vi "Kinect - Control Cluster (SubVI).vi"(7 "error in":errorcluster, 8 "Calibrate Pitch":bool, 9 "Weak detect":bool, 10 "Array of Joint Positions in":dbl[][](array[numeric])=[[-0.1347254365682602, -0.08132069557905197, 1.9283822774887085], [-0.13885043561458588, -0.016961583867669106, 2.011981248855591], [-0.14481712877750397, 0.43931880593299866, 2.1406660079956055], [-0.141028493642807, 0.6465446352958679, 2.1821846961975098], [-0.30089935660362244, 0.32630765438079834, 2.0420639514923096], [-0.26517531275749207, 0.1817575842142105, 1.7472813129425049], [-0.12027974426746368, 0.18339265882968903, 1.4648816585540771], [-0.08502443134784698, 0.17742732167243958, 1.430349588394165], [-0.003267590655013919, 0.3257020115852356, 2.05509090423584], [0.025156527757644653, 0.16852739453315735, 1.7666873931884766], [-0.0971737802028656, 0.17441977560520172, 1.473292350769043], [-0.1705384999513626, 0.18324872851371765, 1.465440034866333], [-0.21323969960212708, -0.14314982295036316, 1.8959753513336182], [-0.2711157202720642, -0.4896538555622101, 1.8643081188201904], [-0.25042033195495605, -0.8901764750480652, 1.868118405342102], [-0.23817336559295654, -0.9496505260467529, 1.7813631296157837], [-0.05292607098817825, -0.14255109429359436, 1.9082472324371338], [-0.03935781121253967, -0.4929194450378418, 1.869278073310852], [-0.03272760659456253, -0.8968366384506226, 1.8476512432098389], [-0.02717301808297634, -0.9465184211730957, 1.7542997598648071]]) -> (0 "error out":errorcluster, 2 "Control Cluster out":T1={"Roll"=0.09503769, "Pitch"=0.11711881, "Vertical Speed"=0.0, "Yaw Speed"=-0.05722916} {"Yaw Speed" scale=-1.0..1.0; "Vertical Speed" scale=-1.0..1.0; "Pitch" scale=-1.0..1.0; "Roll" scale=-1.0..1.0}, 3 "Array of Joint Positions out":dbl[][](array[numeric])=[[-0.1347254365682602, -0.08132069557905197, 1.9283822774887085], [-0.13885043561458588, -0.016961583867669106, 2.011981248855591], [-0.14481712877750397, 0.43931880593299866, 2.1406660079956055], [-0.141028493642807, 0.6465446352958679, 2.1821846961975098], [-0.30089935660362244, 0.32630765438079834, 2.0420639514923096], [-0.26517531275749207, 0.1817575842142105, 1.7472813129425049], [-0.12027974426746368, 0.18339265882968903, 1.4648816585540771], [-0.08502443134784698, 0.17742732167243958, 1.430349588394165], [-0.003267590655013919, 0.3257020115852356, 2.05509090423584], [0.025156527757644653, 0.16852739453315735, 1.7666873931884766], [-0.0971737802028656, 0.17441977560520172, 1.473292350769043], [-0.1705384999513626, 0.18324872851371765, 1.465440034866333], [-0.21323969960212708, -0.14314982295036316, 1.8959753513336182], [-0.2711157202720642, -0.4896538555622101, 1.8643081188201904], [-0.25042033195495605, -0.8901764750480652, 1.868118405342102], [-0.23817336559295654, -0.9496505260467529, 1.7813631296157837], [-0.05292607098817825, -0.14255109429359436, 1.9082472324371338], [-0.03935781121253967, -0.4929194450378418, 1.869278073310852], [-0.03272760659456253, -0.8968366384506226, 1.8476512432098389], [-0.02717301808297634, -0.9465184211730957, 1.7542997598648071]])   [LabVIEW 2014]
uses:
  Resources/Others/Control cluster.ctl
panel:
  out "vertical speed":dbl(knob)=-0.14245328307151794 scale=-20.0..20.0
  in  "pitch offset":dbl=0.15 format="%#_13g"
  in  "roll adjust":dbl=1.5 format="%#_13g"
  # "Experiment-based values:"
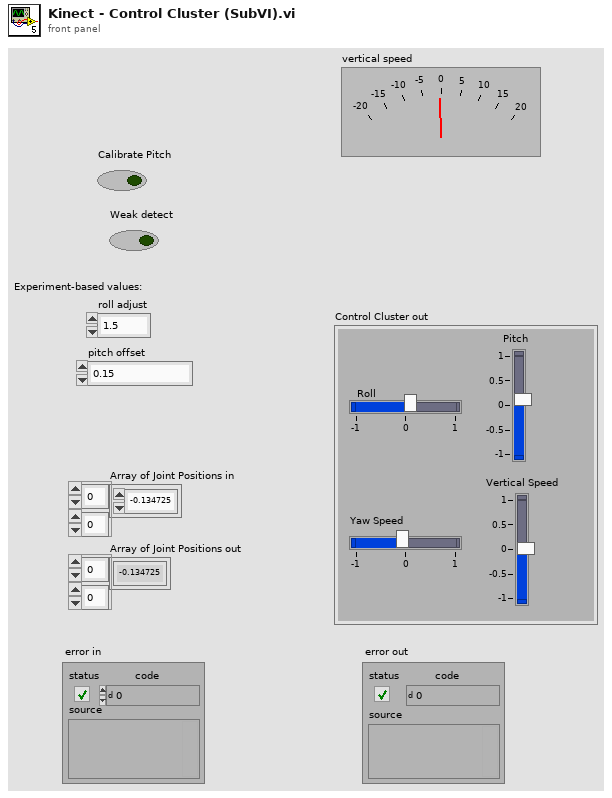
[diagram p1: front panel]
types:
  T1 = typedef "Control cluster.ctl" = cluster{"Roll":sgl, "Pitch":sgl, "Vertical Speed":sgl, "Yaw Speed":sgl}
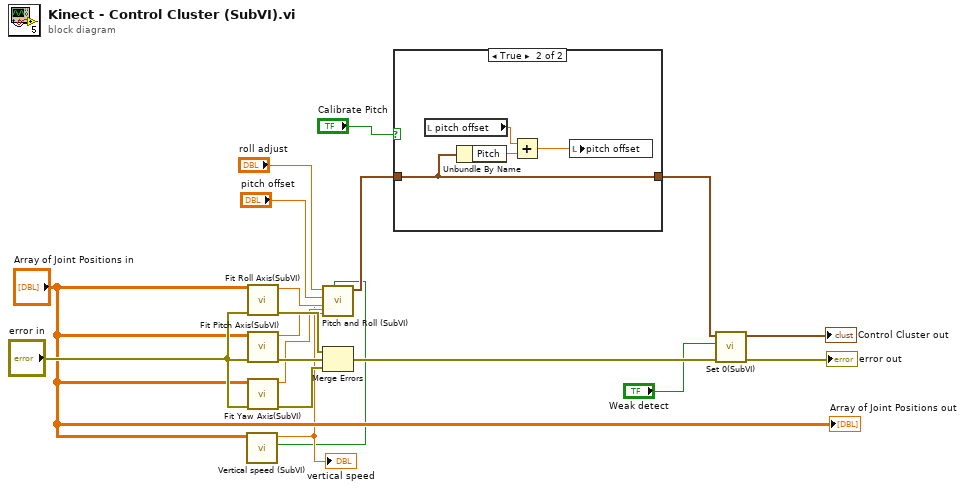
[diagram p0: block diagram]
diagram:
  n1 = call "Vertical speed (SubVI).vi"("Array of Joint Positions in"="Array of Joint Positions in") -> ("x .and. y?"=w1:bool, "Vertical Speed"=w2:dbl)  [unwired: 9 in]
  "vertical speed" <- w2
  n2 = call "Fit Roll Axis(SubVI).vi"("error in (no error)"="error in", "Array of Joint Positions in"="Array of Joint Positions in") -> ("error out"=w18:errorcluster, "slope"=w19:dbl)  [unwired: 8 in]
  n3 = call "Fit Pitch Axis(SubVI).vi"("error in (no error)"="error in", "Array of Joint Positions in"="Array of Joint Positions in") -> ("error out"=w17:errorcluster, "slope"=w16:dbl)  [unwired: 8 in]
  n4 = call "Fit Yaw Axis(SubVI).vi"("error in (no error)"="error in", "Array of Joint Positions in in"="Array of Joint Positions in") -> ("error out"=w11:errorcluster, "slope"=w12:dbl)  [unwired: 8 in]
  n5 = call "Pitch and Roll (SubVI).vi"("Vertical Speed"=w2, "yaw"=w12, "Vertical movement"=w1, "pitch"=w16, "roll"=w19, "pitch offset"="pitch offset", "roll adjust"="roll adjust") -> ("Control Cluster out"=w5:T1)  [unwired: 2 in]
  n6 = Merge Errors(w18, w17, w11) -> (w10:errorcluster)
  n7 = case shown="True" "Calibrate Pitch" {
    tunnel: w5 -> [w20 w24]
    tunnel: [w20 w24] -> w4
    frame False {
    }
    frame True {
      n8 = local read "pitch offset"() -> (w23:dbl)
      n9 = Unbundle By Name(w24) -> ("Pitch"=w22:sgl)
      n10 = Add(x=w23, y=w22) -> (x+y=w21:dbl)
      n11 = local write "pitch offset"(w21) -> ()
    }
  }
  n12 = call "Set 0(SubVI).vi"("error in (no error)"=w10, "Weak detect"="Weak detect", "Control Cluster in"=w4) -> ("error out"=→"error out":errorcluster, "Control Cluster out"=→"Control Cluster out":T1)  [unwired: 7 in]
  "Array of Joint Positions out" <- "Array of Joint Positions in"
